vi "E816_Sample_Application_1a.vi"() -> ()   [LabVIEW 2011]
doc: "This VI demonstrates how to initialize an E-816 system with more than one axis, how to move all connected axes and how to query for the position value. \n\nIn this example the E-816 is connected through COM port 1 with baudrate 57600. The VI runs E816_Configuration_Setup.vi with specified settings, moves the connected axes relative to their current position, waits for the movement to finish and reads the position of the axes and the error status of the controller. Instead of calling the corresponding command VIs, it uses \"Split multiple axes command.vi\" which sends the chosen commands for the given axes one after another and returns the answer array (if any). The diagram shows how to combine the driver VIs for these tasks. \n\nFor an example of how to command a single axis E-816 system see E816_Sample_ Application_1.vi\n\nWarning: Before running this VI, modify the \"RS232 settings\" on the block diagram to reflect your configuration. The predefined settings provided with the VI probably do not match your system."
panel:
  in  "stop":bool
  in  "error in":errorcluster
  out "Running":bool caption="Configuration_Setup.vi is running"
  out "error out":errorcluster
  out "Position":dbl[](array[numeric]) format="%.6f"
  out "Conn. Axes":string[](array[string])
  out "Identification":string
  # "This VI demonstrates how to initialize an E-816 system with more than one axis, how to move all connected axes and how to query\nfor the position value. The VI runs E816_Configuration_Setup.vi with specified settings, moves the connected axes relative to their \ncurrent position and reads the position. Instead of calling the corresponding command VIs, it uses \"Split multiple axes command.vi\"\nwhich sends the chosen commands for the given axes one after another and returns the answer array (if any). The diagram shows\nhow to combine the driver VIs for these tasks. \n\nWarning: Before running this VI, modify the interface settings on the block diagram to reflect your configuration. The predefined \n                 settings provided with the VI probably do not match your system."
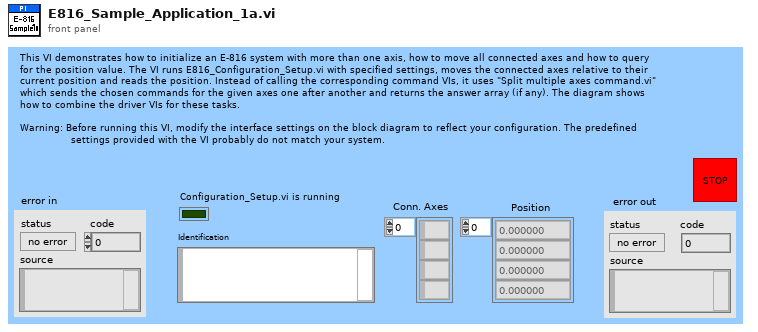
[diagram p1: front panel]
types:
  T1 = enum16{"DCO", "DCO?", "MOV", "MOV?", "MVR", "ONT?", "OVF?", "POS?", "RST", "SVA", "SVA?", "SVO", "SVO?", "SVR", "VOL?", "GWait"}
  T2 = enum16{"DCO", "DCO?", "MOV", "MOV?", "MVR", "ONT?", "OVF?", "POS?", "RST", "SVA", "SVA?", "SVO", "SVO?", "SVR", "VOL?"}
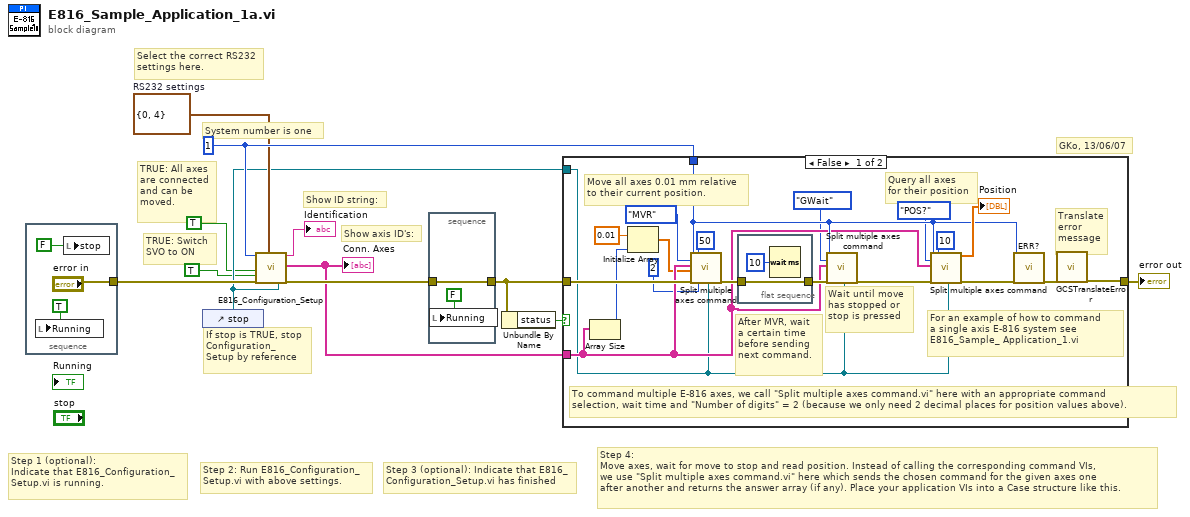
[diagram p0: block diagram]
diagram:
  w4 = cluster{"Portnumber":i32, "Baudrate":u16} {"Portnumber"=0, "Baudrate"=4}  # RS232 settings
  w8 = 1 ("System no.")
  # "TRUE: All axes\nare connected\nand can be\nmoved."
  # "TRUE: Switch\nSVO to ON"
  # "If stop is TRUE, stop\nConfiguration_\nSetup by reference"
  # "Step 4: \nMove axes, wait for move to stop and read position. Instead of calling the corresponding command VIs,\nwe use \"Split multiple axes command.vi\" here which sends the chosen command for the given axes one\nafter another and returns the answer array (if any). Place your application VIs into a Case structure like this."
  # "Select the correct RS232\nsettings here."
  # "GKo, 13/06/07"
  # "Step 3 (optional): Indicate that E816_\nConfiguration_Setup.vi has finished"
  # "Step 2: Run E816_Configuration_\nSetup.vi with above settings."
  # "Step 1 (optional): \nIndicate that E816_Configuration_\nSetup.vi is running."
  # "Show axis ID's:"
  # "Show ID string:"
  # "System number is one"
  n1 = stacked-sequence {
    tunnel: ["error in"] -> w9
    frame #0 {
      n2 = local write "Running"(TRUE ("Running")) -> ()
      n3 = local write "stop"(FALSE ("stop")) -> ()
    }
  }
  n4 = control-ref of="stop"() -> (w3:refnum<vi>)
  n5 = call "E816_Configuration_Setup.vi"("System no."=w8, "All axes?"=TRUE, "Change servo \nstatus to ON?"=TRUE ("Use dialog to define\nconnected stages?"), "error in"=w9, "RS232 settings"=w4, "Stop refnum"=w3) -> ("Identification"=→"Identification":string, "Conn. Axes"=w5:string[], "error out"=w10:errorcluster)  [unwired: 10 in, 1 out]
  "Conn. Axes" <- w5
  n6 = stacked-sequence {
    tunnel: w10 -> [w17]
    tunnel: [w17] -> w7
    frame #0 {
      n7 = local write "Running"(FALSE ("Running")) -> ()
    }
  }
  n8 = Unbundle By Name(w7) -> ("status"=w6:bool)
  n9 = case shown="False" w6 {
    tunnel: [w35 w40] -> w11
    tunnel: w5 -> [w28 _]
    tunnel: w8 -> [w32 _]
    tunnel: w7 -> [w36 w40]
    tunnel: w3 -> [w20 _]
    frame False {
      # "For an example of how to command\na single axis E-816 system see \nE816_Sample_ Application_1.vi"
      # "After MVR, wait\na certain time\nbefore sending\nnext command."
      # "Translate\nerror \nmessage"
      # "Wait until move\nhas stopped or\nstop is pressed"
      # "Query all axes\nfor their position"
      # "To command multiple E-816 axes, we call \"Split multiple axes command.vi\" here with an appropriate command\nselection, wait time and \"Number of digits\" = 2 (because we only need 2 decimal places for position values above)."
      # "Move all axes 0.01 mm relative\nto their current position."
      n10 = Array Size(array=w28) -> (size(s)=w27:i32)
      n11 = Initialize Array(0.01 ("Numeric"), w27) -> (w25:dbl[])
      n12 = call "Split multiple axes command.vi"("System no."=w32, "Command"=T2."MVR", "Axes to command"=w28, "Num. values in"=w25, "error in"=w36, "Wait time (ms)"=u32 50, "No.of digits"=i16 2, "Stop refnum"=w20) -> ("error out"=w30:errorcluster)  [unwired: 9 in, 2 out]
      n13 = flat-sequence {
        tunnel: w30 -> [w39]
        tunnel: [w39] -> w29
        frame #0 {
          n14 = Wait (ms)(milliseconds to wait=u32 10) -> ()  [unwired: 1 out]
        }
      }
      n15 = call "Split multiple axes command.vi"("System no."=w32, "Command"=T1."GWait", "Axes to command"=w28, "error in"=w29, "Stop refnum"=w20) -> ("error out"=w31:errorcluster)  [unwired: 12 in, 2 out]
      n16 = call "Split multiple axes command.vi"("System no."=w32, "Command"=T2."POS?", "Axes to command"=w28, "error in"=w31, "Wait time (ms)"=u32 10, "Stop refnum"=w20) -> ("Num. values out"=→"Position":dbl[], "error out"=w34:errorcluster)  [unwired: 11 in, 1 out]
      n17 = call "ERR?.vi"("System no."=w32, "error in"=w34) -> ("error out"=w33:errorcluster)  [unwired: 16 in, 1 out]
      n18 = call "GCSTranslateError.vi"("error in"=w33) -> ("error out"=w35:errorcluster)  [unwired: 16 in, 2 out]
    }
    frame True {
      # "Error during initialization"
    }
  }
  "error out" <- w11
